vi "Pcre2PatternInfoBytes8.vi"(8 "error in":errorcluster, 10 "What":u32 format="%.0x", 11 "pCode":u64 format="%.0x") -> (0 "error out":errorcluster, 2 "DataBytes":u8[](array[numeric]) format="%02x", 3 "pCode":u64 format="%.0x")   [LabVIEW 2021, in "libpcre2-8.lvlib"]
uses:
  libpcre2-8.lvlib
  <vilib>/Utility/error.llb/Error Cluster From Error Code.vi
  libpcre2-8-x32.dll
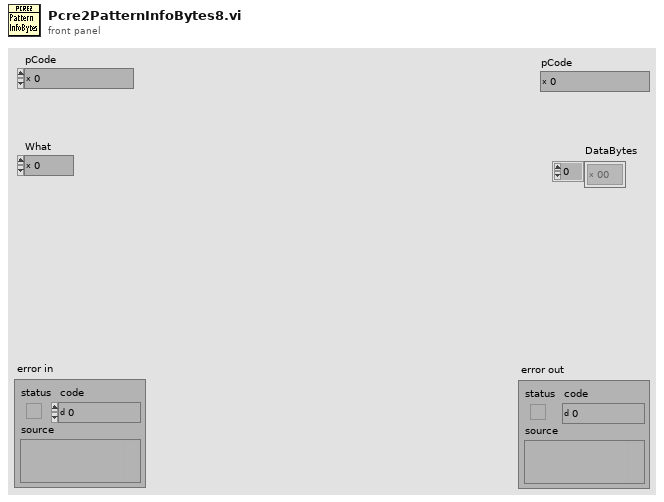
[diagram p1: front panel]
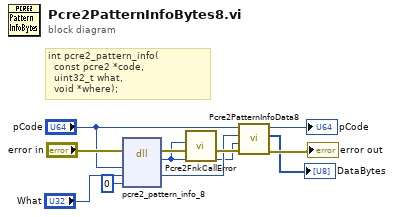
[diagram p0: block diagram]
diagram:
  # "int pcre2_pattern_info(\n  const pcre2 *code,\n  uint32_t what,\n  void *where);"
  n1 = dll-call lib="libpcre2-8-x*.dll" fn="pcre2_pattern_info_8"(error in="error in", "code"="pCode", "what"="What", "where"=u64 0) -> (error out=w8:errorcluster, "return type"=w1:i32, "what"=w2:u32)  [unwired: 4 in, 1 out]
  n2 = call "Pcre2FnkCallError.vi"("error in"=w8, "ErrorCode"=w1) -> ("error out"=w7:errorcluster)  [unwired: 9 in]
  n3 = call "Pcre2PatternInfoData8.vi"("error in"=w7, "size"=w1, "What"=w2, "pCode"="pCode") -> ("error out"=→"error out":errorcluster, "DataBytes"=→"DataBytes":u8[], "pCode"=→"pCode":u64)  [unwired: 5 in]
